vi "Out_S7F20.vi"(8 "error in (no error)":errorcluster, 10 "PPID":string[](array[string]), 11 "S7 Message Class in":refnum<class "S7 Message Class.lvclass">) -> (0 "error out":errorcluster, 3 "S7 Message Class out":refnum<class "S7 Message Class.lvclass">)   [LabVIEW 2020, in "SECS Communication.lvlib" / "S7 Message Class.lvclass"]
uses:
  S7 Message Class.lvclass
  D:/Dropbox/SECS/LabVIEW Code/Com/SECS Communication/SECS-II Class/SECS-II Class.lvclass
  SECS-II Class/Data Message_List.vi
  SECS-II Class/Data Message_ASCII.vi
  S7 Message Class.lvclass/S7 Message Class.ctl
  SECS-II Class/SECS-II Class.lvclass
  D:/Dropbox/SECS/LabVIEW Code/Com/SECS Communication/S7 Message Class/S7 Message Class.lvclass
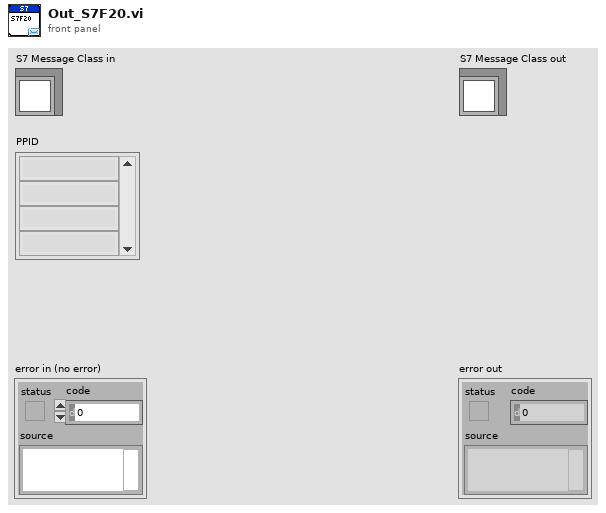
[diagram p1: front panel]
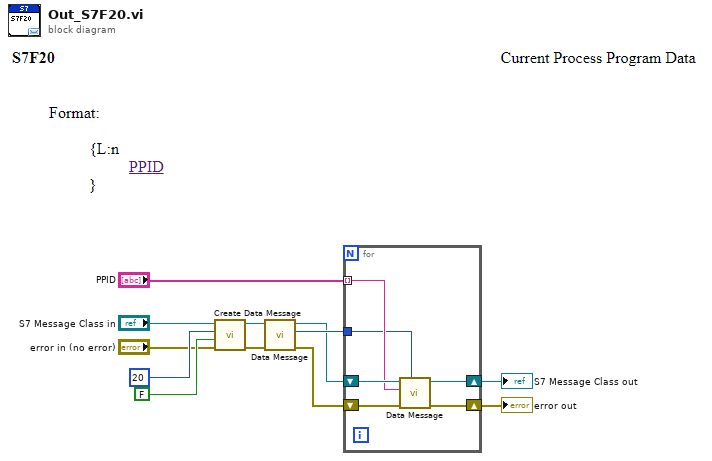
[diagram p0: block diagram]
diagram:
  n1 = call "Create Data Message.vi"("error in (no error)"="error in (no error)", "W-Bit"=FALSE, "Function"=u8 20, "SECS-II Class in"="S7 Message Class in") -> ("error out"=w7:errorcluster, "SECS-II Class out"=w8:refnum<class "S7 Message Class.lvclass">)  [unwired: 6 in]
  n2 = call-poly "Data Message.vi"("error in"=w7, "SECS-II Class in"=w8) -> ("error out"=w6:errorcluster, "Index"=w5:i32, "SECS-II Class out"=w4:refnum<class "S7 Message Class.lvclass">)  [unwired: 7 in]
  n3 = for {
    tunnel: w5 -> [w15]
    shift-right: [w13] -> w1
    shift-left: w6 -> [w18]
    shift-right: [w14] -> w2
    shift-left: w4 -> [w17]
    tunnel: "PPID" -> [w16] mode=indexing
    n4 = call-poly "Data Message.vi"("Parent Index"=w15, "error in"=w18, "Data"=w16, "SECS-II Class in"=w17) -> ("error out"=w13:errorcluster, "SECS-II Class out"=w14:refnum<class "S7 Message Class.lvclass">)  [unwired: 6 in]
  }
  "error out" <- w1
  "S7 Message Class out" <- w2
